vi "HEWH Event Lead Check.vi"(8 "error in (no error)":errorcluster, 10 "Power State":T1) -> (0 "error out":errorcluster, 1 "Comp":i16, 2 "LE":i16, 3 "UE":i16, 4 "Fans":i16)   [LabVIEW 2023]
uses:
  Type Definitions/HEWH Power Elements.ctl
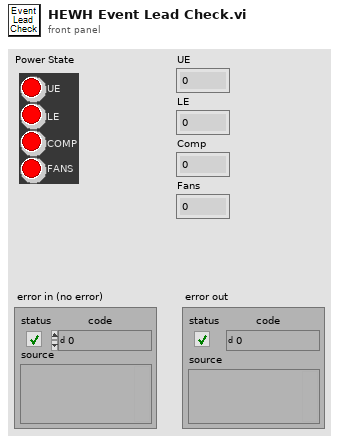
[diagram p1: front panel]
types:
  T1 = typedef "HEWH Power Elements.ctl" = cluster{"UE":bool, "LE":bool, "COMP":bool, "FANS":bool}
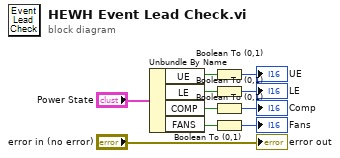
[diagram p0: block diagram]
diagram:
  n1 = Unbundle By Name("Power State") -> ("UE"=w4:bool, "LE"=w3:bool, "COMP"=w2:bool, "FANS"=w1:bool)
  n2 = Boolean To (0,1)(Boolean=w4) -> (0, 1=→"UE":i16)
  n3 = Boolean To (0,1)(Boolean=w3) -> (0, 1=→"LE":i16)
  n4 = Boolean To (0,1)(Boolean=w2) -> (0, 1=→"Comp":i16)
  n5 = Boolean To (0,1)(Boolean=w1) -> (0, 1=→"Fans":i16)
  "error out" <- "error in (no error)"
